vi "sendOutputData.vi"(8 "error in (no error)":errorcluster, 9 "outputData":T1 {"Step & Direction" min=-32767}, 10 "model":refnum<class "Model.lvclass">, 11 "DataOnDemandState in":refnum<class "DataOnDemandState.lvclass">) -> (0 "error out":errorcluster, 2 "model 2":refnum<class "Model.lvclass">, 3 "DataOnDemandState out":refnum<class "DataOnDemandState.lvclass">)   [LabVIEW 2013, in "DataOnDemandState.lvclass"]
uses:
  DataOnDemandState.lvclass
  Model/Model/Model.lvclass
  <userlib>/Common/ILC/Typedefs/OutputData.ctl
  Model/Model/Model.lvclass/Model.ctl
  <userlib>/Common/ILC/Typedefs/ILCTypedefs.lvlib
panel:
  # "DAC"
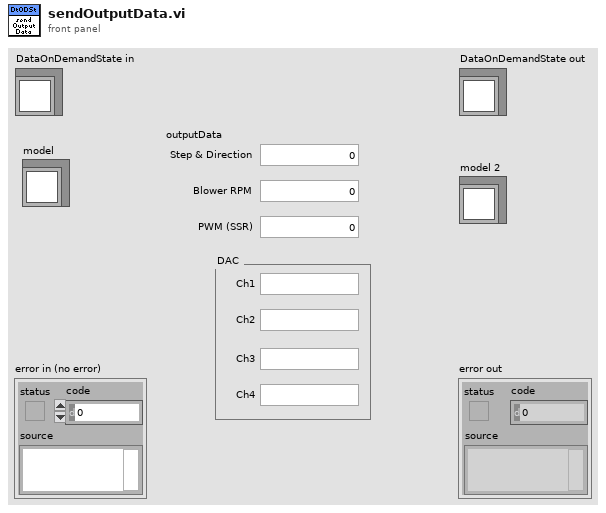
[diagram p1: front panel]
types:
  T1 = typedef "ILCCommon.lvlib/ILCTypedefs.lvlib/OutputData.ctl" = cluster{"Step & Direction":i16, "Blower RPM":u8, "PWM (SSR)":u8, "Ch1":u16, "Ch2":u16, "Ch3":u16, "Ch4":u16}
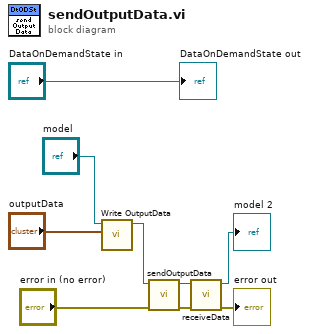
[diagram p0: block diagram]
diagram:
  n1 = call "Write OutputData.vi"("OutputData"="outputData", "Model in"="model") -> ("Model out"=w1:refnum<class "Model.lvclass">)  [unwired: 9 in]
  n2 = call "sendOutputData.vi"("error in (no error)"="error in (no error)", "Model in"=w1) -> ("error out"=w6:errorcluster, "Model out"=w7:refnum<class "Model.lvclass">)  [unwired: 8 in]
  n3 = call "receiveData.vi"("error in (no error)"=w6, "Model in"=w7) -> ("error out"=→"error out":errorcluster, "Model out"=→"model 2":refnum<class "Model.lvclass">)  [unwired: 8 in]
  "DataOnDemandState out" <- "DataOnDemandState in"
